vi "AH2700 Time Test.vi"() -> ()   [LabVIEW 2020]
uses:
  New NML Data Acq/Sub Controls/Instrument Properties.ctl
  New NML Data Acq/Sub Controls/Public.ctl
  New NML Data Acq/Sub Controls/Private.ctl
  New NML Data Acq/Sub Controls/Instrument Ref.ctl
  New NML Data Acq/Sub Controls/SystemCheckBox-resize.ctl
  New NML Data Acq/Sub Controls/Instrument Actions.ctl
  <vilib>/Analysis/NI_AALBase.lvlib
panel:
  out "Histogram Graph":T1(graph)
  out "Freq Index":i32
  out "Data":dbl[](array[numeric]) format="%_10f"
  out "Current Stats":dbl[](array[numeric]) format="%.3f"
  in  "Expected Value":dbl=100.0
  out "Count":i32
  out "Average":i32
  out "Current Frequency":dbl
  out "Array":dbl[][][](array[numeric])=[[[35.680109375, 0.6458252040579002, 35.498, 38.6, 64.0], [35.632625000000004, 0.528468752361218, 35.498, 38.549, 64.0], [35.539093750000006, 0.02657825746434977, 35.497, 35.656, 64.0], [36.008609375000006, 1.1004477100027956, 35.498, 38.6, 64.0], [36.059421875, 1.1460347899742611, 35.499, 38.599, 64.0], [36.01325000000001, 1.1049814334431005, 35.498, 38.601, 64.0], [36.20160937500001, 1.262523293730576, 35.498, 38.709, 64.0], [36.203921875, 1.2531691293737954, 35.498, 38.598, 64.0], [45.552343750000006, 1.1118567656231204, 45.047, 48.151, 64.0], [64.67654687500001, 1.1525081403794388, 64.1, 67.201, 64.0], [102.92346875000004, 1.2293001489265316, 102.249, 105.352, 64.0], [182.00240624999998, 0.9997699690786006, 181.55, 184.701, 64.0], [335.19457812499996, 1.4212888383624092, 334.149, 337.405, 64.0], [640.2555937499998, 1.285364116391284, 639.352, 642.698, 64.0], [1250.9235312499995, 1.329125825242058, 1249.751, 1253.499, 64.0], [2474.9906874999997, 1.2232058435579556, 2473.851, 2477.898, 64.0]], [[34.15467187499999, 1.2112240044837705, 33.349, 36.899, 64.0], [34.137171875, 1.2380397531208522, 33.349, 36.9, 64.0], [34.290296875, 1.3852482635744803, 33.347, 36.902, 64.0], [34.474890625, 1.2692667564221218, 33.347, 36.899, 64.0], [34.287546875000004, 1.3042409813567422, 33.348, 36.9, 64.0], [34.42039062500001, 1.3693168105043347, 33.347, 36.901, 64.0], [34.859515625, 1.4357561250245938, 33.348, 36.9, 64.0], [34.409515625000004, 1.38711379000378, 33.347, 36.9, 64.0], [43.403156249999995, 1.312365176370812, 42.399, 45.951, 64.0], [61.656375, 1.3327292738813536, 60.55, 64.15, 64.0], [98.21567187499998, 1.4193065046412856, 96.85, 100.601, 64.0], [173.53993749999998, 1.4269995258672636, 172.249, 175.851, 64.0], [318.38918749999993, 1.3004074193687212, 317.35, 321.052, 64.0], [609.0055312500001, 1.3376146023443207, 607.85, 611.599, 64.0], [1189.589046875, 1.035762834128312, 1188.749, 1192.4, 64.0], [2354.58440625, 1.292604946078635, 2353.049, 2357.304, 64.0]], [[34.75109375000001, 0.33744698437221915, 32.101, 34.921, 64.0], [34.712625, 0.47329498503274114, 32.1, 34.908, 64.0], [34.79143750000001, 0.02651676618460264, 34.748, 34.904, 64.0], [34.796265625, 0.021375139236528, 34.75, 34.911, 64.0], [34.795375, 0.028151799401171303, 34.748, 34.955, 64.0], [34.79615625000001, 0.022587550124680004, 34.749, 34.904, 64.0], [34.796921874999995, 0.025438568822364106, 34.749, 34.954, 64.0], [34.639984375000004, 0.6694339587657692, 32.051, 35.448, 64.0], [43.42746875, 0.6550800258577406, 40.899, 43.71, 64.0], [61.212609374999985, 0.029894851278045725, 61.148, 61.355, 64.0], [96.28523437499999, 0.6603404062549382, 93.749, 96.555, 64.0], [169.3985625, 0.6514420603065991, 166.899, 169.709, 64.0], [310.4539375, 0.07490520464253225, 310.3, 310.701, 64.0], [592.28128125, 0.06330286704557714, 592.101, 592.4, 64.0], [1155.7351875000002, 0.6178266535279325, 1153.301, 1156.301, 64.0], [2285.9500468749998, 0.3492272389641416, 2284.099, 2286.65, 64.0]], [[22.389156250000006, 0.026679888835112388, 22.347, 22.507, 64.0], [22.38890625000001, 0.0254238475414227, 22.347, 22.49, 64.0], [22.3896875, 0.029155780281267054, 22.347, 22.541, 64.0], [22.374859375000007, 0.08089830323480102, 21.95, 22.49, 64.0], [22.381375000000006, 0.06112061975086742, 21.949, 22.509, 64.0], [22.389921875000006, 0.025948853653916363, 22.348, 22.506, 64.0], [22.389156250000006, 0.026304818045007186, 22.347, 22.505, 64.0], [22.390671875, 0.025355913926177833, 22.348, 22.504, 64.0], [27.756406250000005, 0.025326263894564844, 27.7, 27.909, 64.0], [38.48835937500001, 0.026896844204750057, 38.448, 38.607, 64.0], [59.946937499999976, 0.07976928537281043, 59.499, 60.053, 64.0], [104.645328125, 0.06465538799225248, 104.201, 104.802, 64.0], [190.512546875, 0.03926625825945579, 190.448, 190.605, 64.0], [362.23907812500005, 0.0591844854958851, 362.102, 362.455, 64.0], [705.7094218749999, 0.0946466787563285, 705.449, 705.95, 64.0], [1394.2602031249999, 0.1881717536692792, 1393.899, 1394.75, 64.0]], [[20.119749999999996, 0.029883371178899207, 20.098, 20.262, 64.0], [20.118015624999998, 0.029038831247797867, 20.098, 20.254, 64.0], [20.119578125, 0.029699983799631628, 20.098, 20.255, 64.0], [20.121171874999998, 0.030004525948278734, 20.098, 20.256, 64.0], [20.12115625, 0.02950341317354455, 20.098, 20.254, 64.0], [20.118812499999994, 0.029183532538549214, 20.098, 20.253, 64.0], [20.121234374999997, 0.029925697502844035, 20.098, 20.26, 64.0], [20.11967187499999, 0.02985470353918612, 20.097, 20.26, 64.0], [25.024343749999996, 0.030163690329362818, 24.998, 25.156, 64.0], [34.832078125, 0.029021778733789375, 34.797, 34.954, 64.0], [54.45631249999998, 0.023024400445462147, 54.4, 54.553, 64.0], [95.23209375, 0.03525135086908385, 95.198, 95.404, 64.0], [173.71884375000002, 0.03747770501265849, 173.649, 173.807, 64.0], [330.65318749999994, 0.07354490583720144, 330.5, 330.803, 64.0], [644.43759375, 0.08689561677257476, 644.199, 644.658, 64.0], [1273.8344218750003, 0.2717127804676283, 1273.399, 1274.5, 64.0]], [[18.921562500000007, 0.02916775508173293, 18.888, 19.045, 64.0], [18.92150000000001, 0.028069641285644972, 18.898, 19.029, 64.0], [18.920703125000006, 0.027607613217003904, 18.898, 19.026, 64.0], [18.919921875000007, 0.027401949118196052, 18.898, 19.027, 64.0], [18.919734375000004, 0.030007534602771262, 18.898, 19.063, 64.0], [18.919671875, 0.029895083572811884, 18.898, 19.059, 64.0], [18.922000000000004, 0.030370202606324805, 18.898, 19.061, 64.0], [18.922859375000005, 0.030409306839524218, 18.898, 19.065, 64.0], [23.59, 0.027528916975450828, 23.548, 23.708, 64.0], [32.920515625, 0.03006289290407536, 32.898, 33.063, 64.0], [51.586828125, 0.027497506200057656, 51.548, 51.708, 64.0], [90.39075000000003, 0.036751849105840804, 90.348, 90.509, 64.0], [165.07832812500004, 0.041492035834583225, 164.998, 165.215, 64.0], [314.43070312500015, 0.05431614676689691, 314.348, 314.563, 64.0], [613.248578125, 0.12163043226746312, 613.048, 613.698, 64.0], [1212.055546875, 0.14712827031738435, 1211.749, 1212.35, 64.0]], [[17.816656249999998, 0.0295286886329374, 17.798, 17.965, 64.0], [17.817718749999997, 0.027549936623094604, 17.798, 17.934, 64.0], [17.817734374999993, 0.027530786338726063, 17.798, 17.935, 64.0], [17.81534375, 0.026946872333750548, 17.797, 17.935, 64.0], [17.815828124999996, 0.029024649998573397, 17.797, 17.962, 64.0], [17.815812499999996, 0.028893276528829944, 17.798, 17.962, 64.0], [17.81584375, 0.02919024557121701, 17.798, 17.963, 64.0], [17.818875, 0.02945402659297535, 17.798, 17.96, 64.0], [22.257953124999997, 0.023033743148101055, 22.201, 22.36, 64.0], [31.12675, 0.030695121374421677, 31.098, 31.263, 64.0], [48.867406249999995, 0.029459533046225145, 48.846, 49.013, 64.0], [85.71968749999999, 0.03148538335608076, 85.649, 85.863, 64.0], [156.70874999999998, 0.040979669756274886, 156.648, 156.859, 64.0], [298.70846875, 0.06911273715103122, 298.552, 298.989, 64.0], [582.6431093749999, 0.09314029649592803, 582.451, 582.851, 64.0], [1151.900953125, 0.16111480966951955, 1151.549, 1152.201, 64.0]], [[12.034593749999997, 0.028898683855349418, 11.998, 12.164, 64.0], [12.032890624999997, 0.028826859822433472, 11.998, 12.154, 64.0], [12.033609374999997, 0.02827170731533241, 11.998, 12.15, 64.0], [12.032124999999999, 0.029193117257978757, 11.998, 12.158, 64.0], [12.033828124999998, 0.02916812496354362, 11.999, 12.164, 64.0], [12.032171875, 0.029296814219513724, 11.998, 12.157, 64.0], [12.033703124999997, 0.028648210940290315, 11.999, 12.158, 64.0], [12.034593749999997, 0.0289760266262926, 11.998, 12.165, 64.0], [18.054062499999993, 0.019095312314308017, 17.999, 18.157, 64.0], [23.690781250000008, 0.028795650437643813, 23.648, 23.81, 64.0], [37.69114062499999, 0.02669157597772372, 37.649, 37.785, 64.0], [61.56656250000001, 0.030213460156082395, 61.502, 61.709, 64.0], [103.91493750000002, 0.036512609259276095, 103.848, 104.008, 64.0], [194.06262499999997, 0.048098279017490406, 193.949, 194.158, 64.0], [377.20871875, 0.21695939703160655, 375.698, 377.5, 64.0], [736.31140625, 0.1294840455637457, 736.051, 736.651, 64.0]], [[10.913875, 0.026392940374033676, 10.897, 11.04, 64.0], [10.91528125, 0.026391117282687622, 10.898, 11.027, 64.0], [10.913687500000002, 0.025685444584278988, 10.898, 11.026, 64.0], [10.912625000000002, 0.024161822174530907, 10.897, 11.009, 64.0], [10.913406249999996, 0.027790439574537692, 10.897, 11.059, 64.0], [10.915812499999996, 0.02584991787159579, 10.898, 11.011, 64.0], [10.914171874999997, 0.02808747938167244, 10.898, 11.059, 64.0], [10.912640625, 0.027903670571256627, 10.897, 11.06, 64.0], [16.703343750000002, 0.02255308992309843, 16.65, 16.813, 64.0], [21.878234374999998, 0.029866232026758453, 21.848, 22.007, 64.0], [32.232125, 0.030629117798964347, 32.198, 32.358, 64.0], [56.71710937499999, 0.028554663360004038, 56.697, 56.848, 64.0], [95.565765625, 0.034891551798460964, 95.498, 95.661, 64.0], [180.93056249999998, 0.05610106384980118, 180.799, 181.056, 64.0], [343.9290156249999, 0.1001364929099364, 343.65, 344.148, 64.0], [676.3548124999999, 0.11533950919330764, 676.149, 676.75, 64.0]], [[9.85490625, 0.01860339510744764, 9.847, 9.965, 64.0], [9.859046875000002, 0.023257993804144908, 9.847, 9.98, 64.0], [9.856703125000001, 0.021655073592615207, 9.847, 9.982, 64.0], [9.857218749999998, 0.0211183127858414, 9.847, 9.967, 64.0], [9.856406249999997, 0.020395859173581478, 9.847, 9.965, 64.0], [9.855687499999998, 0.019493486905785416, 9.847, 9.967, 64.0], [9.857203125000003, 0.020914170549220915, 9.848, 9.964, 64.0], [9.855625000000002, 0.018946457557238776, 9.847, 9.961, 64.0], [15.229812500000003, 0.029802458085475266, 15.196, 15.36, 64.0], [20.366484375000002, 0.02894164472871517, 20.348, 20.509, 64.0], [30.6329375, 0.029038493882846485, 30.598, 30.758, 64.0], [52.392328124999985, 0.02657248528471503, 52.348, 52.511, 64.0], [93.45318749999998, 0.03566060251073456, 93.398, 93.557, 64.0], [176.92834374999998, 0.05984244359612746, 176.799, 177.053, 64.0], [339.8040468749999, 0.07102725380957979, 339.649, 339.999, 64.0], [669.5345156249999, 0.09183629192149022, 669.3, 669.75, 64.0]], [[5.317374999999999, 0.055725090527389165, 5.05, 5.513, 64.0], [5.275406249999999, 0.12404335119703305, 4.997, 5.426, 64.0], [5.28784375, 0.10080772500475807, 5.047, 5.403, 64.0], [5.2751875, 0.11921847025857052, 5.0, 5.511, 64.0], [5.31890625, 0.07831230087447293, 5.0, 5.411, 64.0], [5.2947187499999995, 0.11687144867705292, 5.0, 5.51, 64.0], [5.31578125, 0.0728051255717879, 5.049, 5.409, 64.0], [5.320437499999998, 0.08153251858799403, 5.0, 5.46, 64.0], [6.464281250000001, 0.1146490114799658, 6.199, 6.712, 64.0], [8.822718749999998, 0.10587420939154965, 8.548, 8.952, 64.0], [13.504781250000002, 0.11398878652034582, 13.247, 13.658, 64.0], [23.254796874999993, 0.0951271796467217, 22.948, 23.548, 64.0], [42.04464062500001, 0.08548598087749393, 41.749, 42.258, 64.0], [79.58610937499998, 0.09248854363846871, 79.299, 79.759, 64.0], [154.7024375, 0.08006284733763569, 154.401, 154.857, 64.0], [305.17040625, 0.17328916275569853, 304.699, 305.602, 64.0]], [[4.787750000000002, 0.02803399297111919, 4.748, 4.917, 64.0], [4.787218749999998, 0.02942705199113371, 4.747, 4.933, 64.0], [4.787218749999999, 0.029322762570431666, 4.748, 4.932, 64.0], [4.786890625, 0.02771688911945777, 4.747, 4.909, 64.0], [4.786796874999998, 0.027499021447236194, 4.748, 4.907, 64.0], [4.786015625, 0.027576440478140854, 4.748, 4.905, 64.0], [4.786875, 0.02786048006058671, 4.747, 4.91, 64.0], [4.787609375000001, 0.027541378501482184, 4.747, 4.908, 64.0], [5.949343750000001, 0.01979756177868758, 5.898, 6.06, 64.0], [8.275203125, 0.030368205850647603, 8.248, 8.412, 64.0], [13.60240625, 0.024902169695742517, 13.547, 13.755, 64.0], [23.221921875000003, 0.029635513170400803, 23.198, 23.352, 64.0], [41.12589062500001, 0.03024404293305624, 41.097, 41.26, 64.0], [78.29778125000001, 0.04687858980963104, 78.248, 78.5, 64.0], [152.65714062499998, 0.04361951914449336, 152.547, 152.751, 64.0], [301.6712031250001, 0.06336845634794074, 301.549, 301.807, 64.0]], [[4.4963750000000005, 0.022037125961316323, 4.449, 4.619, 64.0], [4.495921875000001, 0.024482131279447983, 4.449, 4.637, 64.0], [4.4959218750000005, 0.02442241014035045, 4.449, 4.638, 64.0], [4.496265625, 0.021251511384160676, 4.45, 4.612, 64.0], [4.497, 0.020346209818250017, 4.449, 4.608, 64.0], [4.496249999999999, 0.021433544396502066, 4.448, 4.611, 64.0], [4.495453125, 0.022207484572363132, 4.448, 4.61, 64.0], [4.495515625000001, 0.022266775154782766, 4.448, 4.612, 64.0], [5.552468750000001, 0.019504959686729734, 5.499, 5.659, 64.0], [7.662671874999999, 0.027638858478885763, 7.646, 7.813, 64.0], [11.886078125000001, 0.028300151262986812, 11.847, 12.012, 64.0], [21.574796875, 0.02887695829269627, 21.547, 21.687, 64.0], [37.556453125, 0.029368987902153112, 37.501, 37.664, 64.0], [71.3338125, 0.03879775603067485, 71.251, 71.514, 64.0], [138.95717187499997, 0.04298192853462396, 138.852, 139.108, 64.0], [274.45556250000004, 0.06730453768989665, 274.298, 274.65, 64.0]], [[0.045796874999999994, 0.0009788183270966677, 0.044, 0.048, 64.0], [0.07882812500000003, 0.0023132104228360787, 0.074, 0.082, 64.0], [1.2261875, 0.04771837854321593, 1.149, 1.396, 64.0], [1.4296875, 0.0582051312307369, 1.349, 1.601, 64.0], [2.028171875, 0.07354915313303954, 1.848, 2.202, 64.0], [2.202765625, 0.0065725310712494815, 2.199, 2.253, 64.0], [3.0022968750000003, 0.018688490378279552, 2.997, 3.149, 64.0], [4.52203125, 0.026889526343617985, 4.498, 4.611, 64.0], [7.319671875000001, 0.024660266021235323, 7.298, 7.36, 64.0], [9.907234374999998, 0.017866117784301652, 9.897, 9.963, 64.0], [16.533578125, 0.025463203882939062, 16.497, 16.598, 64.0], [27.401546874999994, 0.017758458469760943, 27.347, 27.451, 64.0], [46.658656249999986, 0.024822684677591956, 46.599, 46.754, 64.0], [88.09312499999999, 0.041037922841086975, 88.048, 88.211, 64.0], [170.98215625, 0.04138177604802538, 170.9, 171.1, 64.0], [337.23678125000004, 0.06379791227862742, 337.099, 337.35, 64.0]], [[0.04460937499999999, 0.0022226624068002712, 0.039, 0.05, 64.0], [0.075875, 0.002200288581361511, 0.073, 0.082, 64.0], [1.2364375, 0.05530058554757592, 1.14, 1.357, 64.0], [1.445046875, 0.054552269877701, 1.348, 1.585, 64.0], [1.95403125, 0.07693967307995785, 1.798, 2.052, 64.0], [2.7555781250000004, 0.022627981475043704, 2.747, 2.906, 64.0], [2.9597812500000003, 0.023547634094077705, 2.948, 3.076, 64.0], [4.47128125, 0.027028772881728565, 4.448, 4.564, 64.0], [7.263437499999999, 0.02258730855893437, 7.248, 7.311, 64.0], [9.843906250000002, 0.01943382646601315, 9.798, 9.908, 64.0], [15.005609374999999, 0.016058046677452375, 14.998, 15.058, 64.0], [27.232859374999997, 0.02563533473361988, 27.198, 27.302, 64.0], [46.445546875000005, 0.02648505399876413, 46.398, 46.549, 64.0], [87.699328125, 0.04146295140587197, 87.648, 87.899, 64.0], [170.24621875000003, 0.06976092251055598, 170.1, 170.5, 64.0], [335.7454218750001, 0.07148311037891743, 335.551, 335.902, 64.0]], [[0.04279687499999999, 0.0009116475143805235, 0.041, 0.045, 64.0], [0.07453125000000001, 0.0017903511227848965, 0.07, 0.08, 64.0], [1.13803125, 0.04628310698368781, 1.08, 1.238, 64.0], [1.4262656249999996, 0.06696273357989548, 1.299, 1.551, 64.0], [1.9219843749999999, 0.08635410527598483, 1.749, 2.057, 64.0], [2.7156562500000003, 0.028373483457130606, 2.698, 2.853, 64.0], [3.5164687499999996, 0.02844765103143578, 3.497, 3.655, 64.0], [4.685671875, 0.026589205762775917, 4.647, 4.784, 64.0], [7.624375, 0.025285355570946782, 7.598, 7.661, 64.0], [10.194671875, 0.018587463506438362, 10.149, 10.259, 64.0], [15.3345625, 0.02561179973594774, 15.297, 15.412, 64.0], [26.105640625, 0.022871183218745043, 26.048, 26.16, 64.0], [46.674343750000006, 0.02669356901922447, 46.647, 46.748, 64.0], [87.78531250000002, 0.029304030277015447, 87.702, 87.853, 64.0], [169.98764062499998, 0.0643093632096331, 169.851, 170.201, 64.0], [334.9305625, 0.09108288132157924, 334.75, 335.2, 64.0]], [[0.04143749999999999, 0.000833333333333333, 0.04, 0.043, 64.0], [0.07156250000000004, 0.0022947490093413263, 0.068, 0.076, 64.0], [1.076640625, 0.019271961035215307, 1.064, 1.167, 64.0], [1.3071718749999999, 0.0381856595236218, 1.199, 1.407, 64.0], [1.8758750000000002, 0.061556142911643935, 1.702, 2.001, 64.0], [2.6616875000000007, 0.02638053334719638, 2.648, 2.8, 64.0], [3.46184375, 0.02707732534093881, 3.447, 3.609, 64.0], [4.631421874999999, 0.02970425905408825, 4.597, 4.763, 64.0], [7.5618437499999995, 0.021589399772566187, 7.548, 7.611, 64.0], [10.122812500000002, 0.02548630195421793, 10.098, 10.162, 64.0], [15.240015624999998, 0.022710386538895278, 15.198, 15.31, 64.0], [25.960218750000006, 0.020404223613502987, 25.948, 26.006, 64.0], [46.438406249999986, 0.026144724649231493, 46.398, 46.5, 64.0], [87.3485625, 0.031112634599886134, 87.297, 87.408, 64.0], [169.20246875000004, 0.06788271134832582, 169.098, 169.359, 64.0], [333.4696406250001, 0.11147330340054809, 333.249, 333.751, 64.0]], [[0.0394375, 0.0008886408384057875, 0.037, 0.041, 64.0], [0.060484375, 0.002960009585462816, 0.059, 0.083, 64.0], [0.41979687499999996, 0.4181574921534321, 0.067, 1.028, 64.0], [1.0312500000000002, 0.1205415030943864, 0.338, 1.25, 64.0], [1.1069843750000001, 0.07690305011547652, 0.996, 1.303, 64.0], [1.36771875, 0.010803392691686875, 1.351, 1.446, 64.0], [1.768046875, 0.029313537523520714, 1.748, 1.907, 64.0], [2.810296875, 0.026678378194621214, 2.798, 2.962, 64.0], [3.3626875, 0.028145807999354094, 3.347, 3.514, 64.0], [4.461093750000001, 0.026948344914869877, 4.447, 4.61, 64.0], [6.933703125000001, 0.056644723955405846, 6.75, 7.107, 64.0], [11.458687500000002, 0.0638805619142176, 11.299, 11.609, 64.0], [20.294687500000002, 0.06133537134295151, 20.048, 20.459, 64.0], [37.856359375, 0.07883282838608044, 37.649, 38.059, 64.0], [73.3368125, 0.2120888459382737, 72.849, 73.699, 64.0], [144.37354687500002, 0.11099376926420693, 144.198, 144.65, 64.0]], [[0.03875, 0.0009258200997725524, 0.037, 0.041, 64.0], [0.05954687499999999, 0.0012463239597706572, 0.057, 0.062, 64.0], [0.28712500000000013, 0.36703010126976676, 0.067, 1.095, 64.0], [1.00884375, 0.2712667648977575, 0.124, 1.267, 64.0], [1.1458593749999997, 0.16141456703283263, 0.193, 1.39, 64.0], [1.4290156250000001, 0.06595609222195076, 1.348, 1.599, 64.0], [1.8261250000000002, 0.035505197473314355, 1.75, 1.97, 64.0], [2.9649531250000005, 0.10342107330122702, 2.849, 3.153, 64.0], [3.586109375, 0.07221267469706937, 3.351, 3.758, 64.0], [4.6891875, 0.067257589410663, 4.498, 4.859, 64.0], [6.893109375, 0.06736729864398082, 6.7, 7.058, 64.0], [11.409546875, 0.0711457100152315, 11.199, 11.561, 64.0], [20.20009375, 0.05858346880699643, 20.049, 20.354, 64.0], [37.74307812500002, 0.0814311092005688, 37.548, 37.905, 64.0], [72.81415625000001, 0.08406143232637607, 72.599, 73.0, 64.0], [143.122, 0.09146080780902453, 142.949, 143.349, 64.0]], [[0.039203125000000005, 0.0035642835273715346, 0.036, 0.058, 64.0], [0.05773437499999999, 0.0028241711103113892, 0.056, 0.079, 64.0], [0.21651562500000004, 0.3235569669518727, 0.066, 1.019, 64.0], [0.8624843750000002, 0.3220957657152088, 0.121, 1.176, 64.0], [1.0681875, 0.13232798058024028, 0.17, 1.224, 64.0], [1.4196093750000003, 0.06044901227743477, 1.348, 1.655, 64.0], [1.7612968750000002, 0.041348568500777526, 1.698, 1.881, 64.0], [2.8438593749999996, 0.10782037784652888, 2.598, 3.058, 64.0], [3.3517656250000005, 0.09153709321648688, 3.147, 3.563, 64.0], [4.370421875000002, 0.08218558261690044, 4.101, 4.61, 64.0], [6.350249999999999, 0.08515066013035323, 6.099, 6.517, 64.0], [10.428984374999999, 0.10589564977312817, 10.199, 10.557, 64.0], [18.411140625000005, 0.08429876332435662, 18.198, 18.563, 64.0], [34.31735937500001, 0.09803099075705364, 34.098, 34.511, 64.0], [66.18135937500001, 0.09176909726210403, 65.95, 66.307, 64.0], [129.93446875, 0.13216199400254997, 129.598, 130.202, 64.0]], [[0.037718749999999995, 0.0025289984842489202, 0.035, 0.056, 64.0], [0.05610937500000001, 0.0008929563436954983, 0.054, 0.059, 64.0], [0.375171875, 0.3829513025814242, 0.063, 0.98, 64.0], [0.7453281250000001, 0.330907269161211, 0.12, 1.116, 64.0], [1.0157812499999999, 0.04729222519074423, 0.949, 1.158, 64.0], [1.3915156250000007, 0.035751342382389716, 1.348, 1.557, 64.0], [1.7426562500000007, 0.019440767792989855, 1.732, 1.837, 64.0], [2.8056562499999997, 0.08329641444101997, 2.648, 3.012, 64.0], [3.318906249999999, 0.07777577024053142, 3.15, 3.509, 64.0], [4.331390625, 0.0584673609090291, 4.149, 4.46, 64.0], [6.317328125000001, 0.06414345398005986, 6.148, 6.511, 64.0], [10.397765625000002, 0.07064009882147612, 10.248, 10.559, 64.0], [18.328218749999998, 0.06959211521429691, 18.151, 18.51, 64.0], [34.24776562500001, 0.07327048003150806, 34.099, 34.408, 64.0], [66.00728125, 0.07893567176997879, 65.749, 66.265, 64.0], [129.650125, 0.11174624030463993, 129.451, 129.9, 64.0]], [[0.037265625000000004, 0.0033582033532686436, 0.034, 0.056, 64.0], [0.055125, 0.0013153549825650611, 0.053, 0.059, 64.0], [0.3305624999999999, 0.36865770569493594, 0.062, 0.934, 64.0], [0.6878281249999999, 0.3780662810238732, 0.11, 1.072, 64.0], [0.97025, 0.07404245886169444, 0.797, 1.104, 64.0], [1.1524375000000002, 0.06645439419584312, 1.012, 1.254, 64.0], [1.6931406249999998, 0.04386590938248495, 1.648, 1.861, 64.0], [2.5013906250000004, 0.05567639412798958, 2.447, 2.65, 64.0], [3.3001250000000013, 0.07594954465520734, 3.149, 3.46, 64.0], [4.307953125, 0.07052151077609481, 4.147, 4.497, 64.0], [6.278281250000001, 0.07787178488356604, 6.099, 6.46, 64.0], [10.364234375, 0.072844854093183, 10.198, 10.562, 64.0], [18.28145312499999, 0.07622521552703451, 18.1, 18.414, 64.0], [34.121281249999996, 0.07735538863449484, 33.948, 34.363, 64.0], [65.7501875, 0.0868470421497402, 65.552, 65.951, 64.0], [129.661734375, 0.30290221808404993, 129.049, 130.15, 64.0]], [[0.0360625, 0.0009236745114890851, 0.034, 0.038, 64.0], [0.0545, 0.0008164965809277267, 0.052, 0.058, 64.0], [0.3715625, 0.3776916469273978, 0.061, 0.924, 64.0], [0.6041562500000001, 0.3981545212822031, 0.108, 1.107, 64.0], [0.9742499999999998, 0.05337676802766691, 0.821, 1.104, 64.0], [1.123375, 0.05925181666225751, 0.993, 1.259, 64.0], [1.6516562499999998, 0.04798121945756401, 1.598, 1.91, 64.0], [2.490578125, 0.06359764513148145, 2.398, 2.697, 64.0], [3.276671875, 0.05685376805859325, 3.198, 3.407, 64.0], [4.23925, 0.03799122705748434, 4.15, 4.412, 64.0], [6.217249999999997, 0.046761807778000486, 6.1, 6.407, 64.0], [10.30246875, 0.05330653158407341, 10.199, 10.461, 64.0], [18.257187499999997, 0.0633012136597211, 18.099, 18.409, 64.0], [34.168875, 0.07139283232885828, 34.048, 34.361, 64.0], [65.95253125, 0.0806457998886651, 65.8, 66.262, 64.0], [129.76103125, 0.127245665251894, 129.447, 130.099, 64.0]], [[0.035859375000000006, 0.0010520907001156494, 0.034, 0.038, 64.0], [0.052765625, 0.0009384585047189705, 0.05, 0.055, 64.0], [0.4195781249999999, 0.36543363259468775, 0.061, 0.919, 64.0], [0.1475, 0.1706273206133254, 0.106, 0.968, 64.0], [0.973921875, 0.09009594615679935, 0.81, 1.238, 64.0], [1.16875, 0.11702774057244744, 0.939, 1.539, 64.0], [1.595375, 0.03213142653895982, 1.548, 1.754, 64.0], [2.422062500000001, 0.04284222624008175, 2.348, 2.663, 64.0], [3.268859375, 0.06570759352785811, 3.099, 3.462, 64.0], [4.214921875, 0.07571150437576366, 4.05, 4.362, 64.0], [6.224984375, 0.10113380923821544, 5.999, 6.4, 64.0], [10.257890625000002, 0.08681601000537849, 10.198, 10.557, 64.0], [18.185140625000003, 0.0801658731150706, 18.099, 18.451, 64.0], [34.15160937500001, 0.46394538598907914, 33.949, 37.75, 64.0], [65.817296875, 0.05896183314532537, 65.748, 66.009, 64.0], [129.46579687500002, 0.07363534772460643, 129.3, 129.75, 64.0]], [[0.03492187500000001, 0.0008223984956906737, 0.033, 0.037, 64.0], [0.048859375000000003, 0.000906190132122148, 0.047, 0.051, 64.0], [0.4915312499999999, 0.4735709989763188, 0.053, 1.128, 64.0], [0.4984687499999999, 0.40133230377774914, 0.094, 0.979, 64.0], [0.8445937500000001, 0.30391141768875235, 0.125, 1.276, 64.0], [0.983515625, 0.08167220431905418, 0.826, 1.376, 64.0], [1.1046562500000001, 0.052486799171806875, 0.999, 1.25, 64.0], [1.7495312500000002, 0.030927959688220475, 1.65, 1.924, 64.0], [2.4446875, 0.032039596038116874, 2.35, 2.614, 64.0], [2.9298125, 0.04775861095797196, 2.798, 3.11, 64.0], [3.8899218750000006, 0.05683484977379214, 3.798, 4.061, 64.0], [5.964937499999998, 0.041770679699278106, 5.849, 6.106, 64.0], [9.878250000000001, 0.04334688432808478, 9.798, 10.061, 64.0], [17.732796875000002, 0.03278606928690462, 17.649, 17.859, 64.0], [33.396890625000005, 0.04579287987473907, 33.299, 33.557, 64.0], [64.81414062500001, 0.052618684347485116, 64.65, 64.961, 64.0]], [[0.034562499999999996, 0.0008886408384057861, 0.033, 0.038, 64.0], [0.32259375, 0.4921232172055068, 0.036, 1.306, 58.0], [0.482453125, 0.4753202739703223, 0.051, 1.306, 61.0], [0.491140625, 0.4012747096555264, 0.09, 1.12, 64.0], [0.5685781249999999, 0.38575338798160375, 0.125, 1.038, 64.0], [0.9647968750000001, 0.07795627176526392, 0.777, 1.113, 64.0], [1.12715625, 0.11359063491886046, 0.908, 1.519, 64.0], [1.7391874999999999, 0.031040615993724114, 1.696, 1.909, 64.0], [2.4188437500000006, 0.05083250389643374, 2.347, 2.549, 64.0], [2.926640625, 0.05148997966548813, 2.848, 3.158, 64.0], [3.88290625, 0.05199472462557032, 3.799, 4.063, 64.0], [5.942312500000002, 0.05193123505755636, 5.848, 6.111, 64.0], [9.868812499999999, 0.047211740199852865, 9.751, 10.009, 64.0], [17.697687500000004, 0.03771441347982217, 17.599, 17.858, 64.0], [33.336828125, 0.03784452516966645, 33.248, 33.511, 64.0], [64.647703125, 0.07144310194466734, 64.498, 64.86, 64.0]], [[0.034296875, 0.0008485222916135317, 0.032, 0.036, 64.0], [0.29162499999999997, 0.4902076819354949, 0.019, 1.307, 50.0], [0.4726249999999999, 0.4397943061773672, 0.051, 1.306, 63.0], [0.6356562499999998, 0.36883218616007346, 0.091, 1.132, 64.0], [0.41043750000000007, 0.372063993258371, 0.124, 0.987, 64.0], [0.9902343750000001, 0.14060410955942934, 0.818, 1.54, 64.0], [1.1521406250000001, 0.20133647641724317, 0.94, 1.931, 64.0], [1.7434375000000002, 0.03018928381301645, 1.697, 1.881, 64.0], [2.4345625, 0.03728435349946436, 2.352, 2.612, 64.0], [2.9250624999999997, 0.03710383328504545, 2.848, 3.061, 64.0], [3.901640625, 0.038244562716560807, 3.8, 4.058, 64.0], [5.93765625, 0.04446193976089653, 5.849, 6.113, 64.0], [9.798625, 0.044017492915200115, 9.748, 9.914, 64.0], [17.644671875, 0.04819637564174316, 17.548, 17.748, 64.0], [33.314937500000006, 0.03791128951929587, 33.25, 33.46, 64.0], [64.61264062500001, 0.05483781778955678, 64.4, 64.813, 64.0]], [[0.034156249999999985, 0.0009295629626804749, 0.032, 0.037, 64.0], [0.37470312499999997, 0.536750826872963, 0.025, 1.306, 52.0], [0.36146875, 0.4369580259799034, 0.05, 1.305, 63.0], [0.41892187499999994, 0.3951386457373649, 0.089, 1.25, 64.0], [0.5661875000000001, 0.42557840659357965, 0.027, 1.316, 63.0], [1.0445625, 0.16097164050732368, 0.77, 1.588, 64.0], [1.165859375, 0.21122611574851805, 0.963, 2.11, 64.0], [1.7286249999999999, 0.03152147164399489, 1.698, 1.882, 64.0], [2.4290468750000005, 0.039535569553512645, 2.349, 2.612, 64.0], [2.9220468749999995, 0.034130203394210246, 2.85, 3.063, 64.0], [3.8923125, 0.0427383605244452, 3.797, 4.06, 64.0], [5.923625000000001, 0.051874543409732875, 5.8, 6.113, 64.0], [9.847796875000002, 0.028209071876102297, 9.749, 9.962, 64.0], [17.668843750000008, 0.0502600282183362, 17.549, 17.807, 64.0], [33.28292187500001, 0.05041016044205417, 33.147, 33.457, 64.0], [64.524328125, 0.1156377835061112, 64.349, 64.756, 64.0]], [[0.03425000000000001, 0.0009594972228385659, 0.032, 0.037, 64.0], [0.34709375, 0.5246204287349395, 0.018, 1.306, 53.0], [0.5341250000000001, 0.4468221655413344, 0.052, 1.305, 63.0], [0.40681249999999997, 0.38798133955290925, 0.09, 0.986, 64.0], [0.526734375, 0.3948829138175011, 0.123, 1.257, 64.0], [1.0065625, 0.12163683587330706, 0.85, 1.319, 64.0], [1.121359375, 0.09203404601015865, 0.918, 1.47, 64.0], [1.6511093749999999, 0.03285374863852182, 1.596, 1.772, 64.0], [2.3540312500000002, 0.03785434438593392, 2.298, 2.561, 64.0], [2.8376562499999993, 0.036328841465455855, 2.798, 3.011, 64.0], [3.811, 0.030756080828618436, 3.798, 3.958, 64.0], [5.875125000000001, 0.04570627409955327, 5.799, 6.007, 64.0], [9.797015625, 0.046804046829341375, 9.699, 9.913, 64.0], [17.648531250000005, 0.03464054361445198, 17.552, 17.749, 64.0], [33.214968750000004, 0.07158898752546078, 33.099, 33.409, 64.0], [64.52198437499999, 0.05583066580337122, 64.4, 64.7, 64.0]], [[0.03434374999999999, 0.0010113443826498764, 0.031, 0.037, 64.0], [0.047359375, 0.0008612871043911417, 0.046, 0.05, 64.0], [0.6163437500000001, 0.449449017846137, 0.05, 1.305, 63.0], [0.20310937499999998, 0.2660311544703167, 0.088, 0.926, 64.0], [0.587796875, 0.3999974674398993, 0.121, 1.284, 64.0], [0.971921875, 0.11584873891216808, 0.725, 1.25, 64.0], [1.1726249999999996, 0.19083779366798262, 0.932, 2.172, 64.0], [1.695453125, 0.04207058682492619, 1.597, 1.81, 64.0], [2.3853281250000005, 0.045926115504334356, 2.296, 2.511, 64.0], [2.8728593750000004, 0.04918215807199852, 2.798, 3.012, 64.0], [3.845359375, 0.046197425609404985, 3.798, 4.005, 64.0], [5.896999999999999, 0.04625979089844934, 5.8, 6.011, 64.0], [9.801703125, 0.045940154199318343, 9.699, 9.957, 64.0], [17.573562499999998, 0.04523444220839678, 17.499, 17.754, 64.0], [33.149328125000004, 0.06713787157486586, 33.049, 33.352, 64.0], [64.41103125, 0.07505151008918137, 64.249, 64.658, 64.0]], [[0.034249999999999996, 0.0018430478552727263, 0.032, 0.047, 64.0], [0.32334375000000004, 0.5052640114139921, 0.046, 1.306, 57.0], [0.4938593749999999, 0.4588160009937068, 0.05, 1.125, 64.0], [0.246859375, 0.2997355377814366, 0.089, 0.978, 64.0], [0.655328125, 0.39092422253917336, 0.123, 1.259, 64.0], [0.9609531250000001, 0.10345790182676637, 0.762, 1.235, 64.0], [1.1225781250000002, 0.17450836198525782, 0.893, 1.81, 64.0], [1.6698281249999998, 0.048324155019341355, 1.6, 1.802, 64.0], [2.38684375, 0.048502076129676004, 2.297, 2.558, 64.0], [2.8588281249999996, 0.04393449477744343, 2.798, 3.001, 64.0], [3.823562500000001, 0.06400468112840814, 3.747, 4.161, 64.0], [5.859453125, 0.051471036604356264, 5.797, 6.05, 64.0], [9.766531250000003, 0.050006973720021476, 9.698, 9.907, 64.0], [17.554078125, 0.04870100050714412, 17.498, 17.701, 64.0], [33.148546875, 0.0650579545512835, 33.048, 33.301, 64.0], [64.35553125, 0.07546637404242508, 64.198, 64.607, 64.0]], [[0.034515625, 0.0008907315969346642, 0.033, 0.037, 64.0], [0.3649374999999999, 0.5362591139566648, 0.038, 1.306, 53.0], [0.6037968750000001, 0.4594191702120552, 0.05, 1.093, 64.0], [0.4445781250000001, 0.3924431332654736, 0.089, 1.25, 64.0], [0.665234375, 0.4321997900070555, 0.049, 1.306, 60.0], [0.9970937499999999, 0.15715786409222973, 0.741, 1.337, 64.0], [1.2488281249999997, 0.2925134404556861, 0.89, 2.037, 64.0], [1.7253124999999998, 0.04695383582214233, 1.697, 1.922, 64.0], [2.418109375, 0.035445069143497265, 2.397, 2.561, 64.0], [2.9307343749999997, 0.05072216327427515, 2.849, 3.116, 64.0], [3.9001406249999997, 0.049276952076527464, 3.799, 4.009, 64.0], [5.9368125, 0.04772103958473263, 5.849, 6.099, 64.0], [9.82353125, 0.050169227509389444, 9.749, 9.96, 64.0], [17.583671875, 0.039226673257380315, 17.499, 17.706, 64.0], [33.10329687500001, 0.05189203678930808, 33.049, 33.362, 64.0], [64.258703125, 0.07296719847692917, 64.148, 64.45, 64.0]], [[0.034140624999999994, 0.0008885012795767511, 0.032, 0.037, 64.0], [0.047468750000000004, 0.0010685808717009124, 0.045, 0.05, 64.0], [0.5396093749999998, 0.5011319129694581, 0.05, 1.306, 56.0], [0.5432187500000001, 0.43437839070276485, 0.089, 1.26, 64.0], [0.7524687500000001, 0.31857111382467196, 0.122, 1.17, 64.0], [1.035640625, 0.14474754894846165, 0.802, 1.346, 64.0], [1.25265625, 0.21314941616413383, 0.866, 1.855, 64.0], [1.7620156250000003, 0.038871171913802384, 1.699, 1.923, 64.0], [2.4587343749999997, 0.03657574970208873, 2.399, 2.609, 64.0], [2.9595624999999997, 0.034324259087484474, 2.899, 3.114, 64.0], [3.929046875, 0.029809676540952155, 3.897, 4.059, 64.0], [5.93915625, 0.03864622561089572, 5.853, 6.057, 64.0], [9.826687499999998, 0.0301387663665127, 9.796, 9.959, 64.0], [17.576703124999998, 0.035961036978312926, 17.5, 17.71, 64.0], [33.071234374999996, 0.03920185539320605, 32.998, 33.208, 64.0], [64.17823437499999, 0.04647810277645133, 64.051, 64.356, 64.0]]] format="%.3g"
  in  "# Calls":i32=64
  out "Data":dbl[](array[numeric]) format="%_10f"
  # "Average"
  # "Std Dev"
  # "Min"
  # "Max"
  # "# Valid"
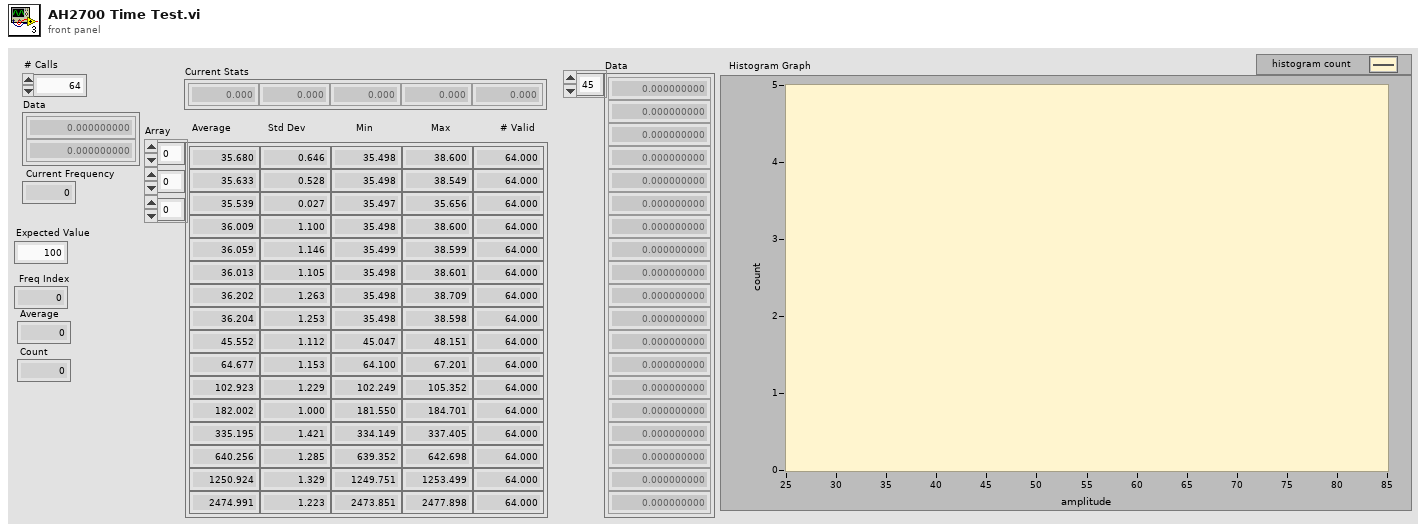
[diagram p1: front panel]
types:
  T1 = cluster{"X Values":dbl[], "Histogram: h(x)":i32[]}
  T2 = typedef "Instrument Properties.ctl" = cluster{"Public":T3, "Private":T4}
  T3 = typedef "Public.ctl" = cluster{"Column Name":string[], "Trace Color":u32[]}
  T4 = typedef "Private.ctl" = cluster{"Path":path, "VI Refnum":T5, "Name":string, "# of Values":i32, "Scale Factors":dbl[], "Display":T6[], "Offset":dbl[]}
  T5 = typedef "Instrument Ref.ctl" = refnum<vi>
  T6 = typedef "SystemCheckBox-resize.ctl" = bool
  T7 = typedef "Instrument Actions.ctl" = enum16{"Scan", "Identify", "New", "Configure", "Initialize", "Test", "Read", "Close"}
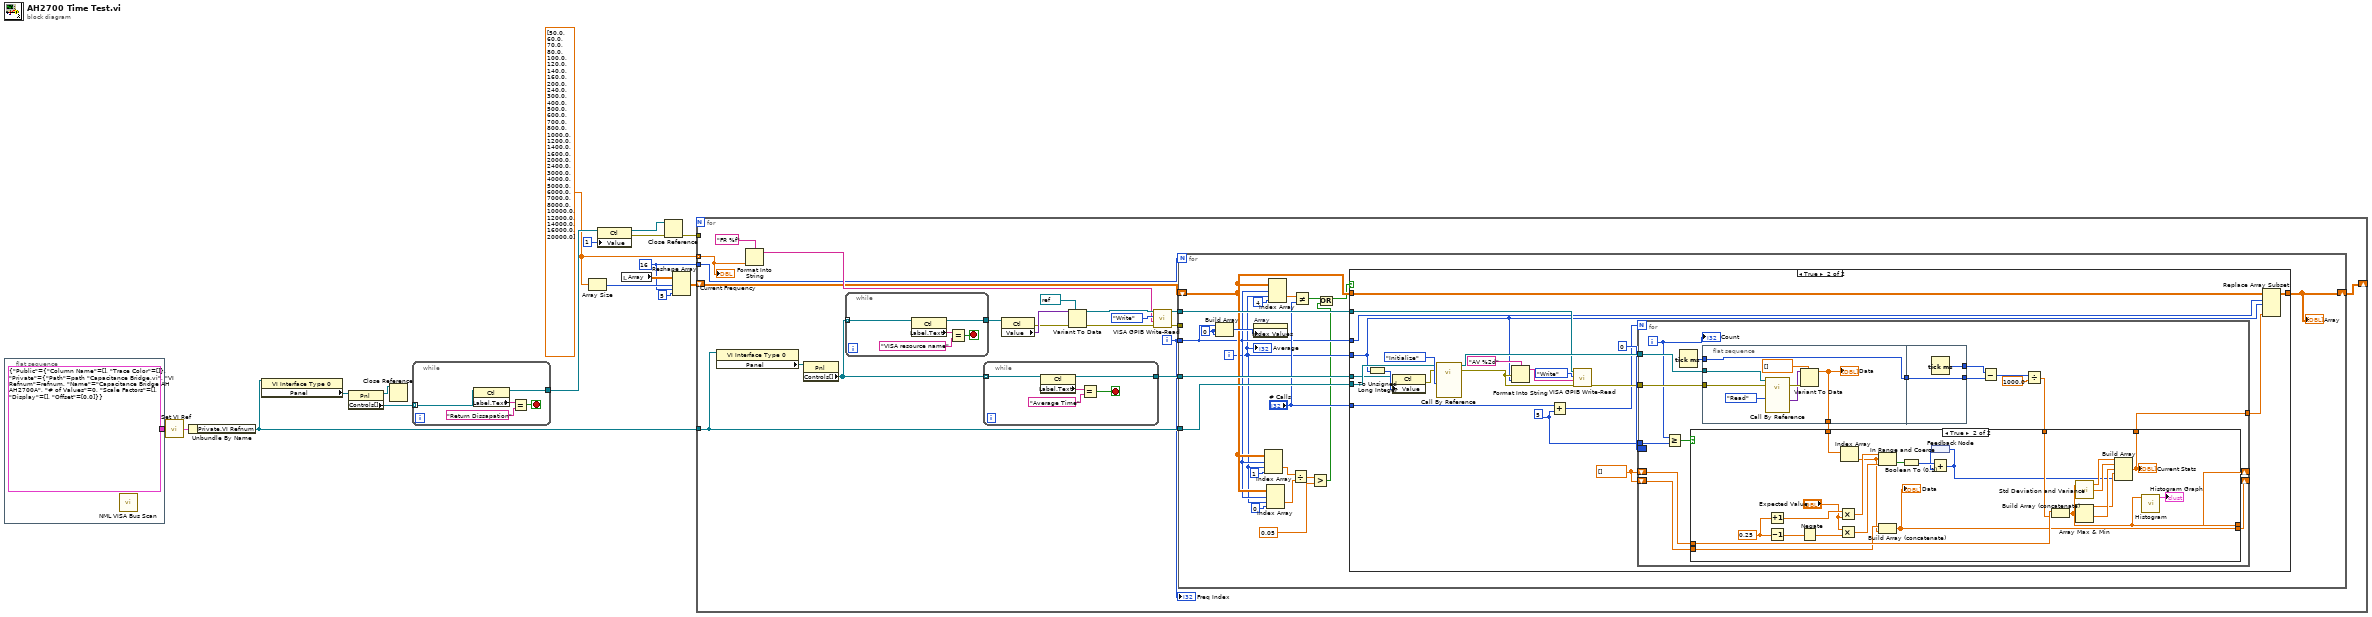
[diagram p0: block diagram]
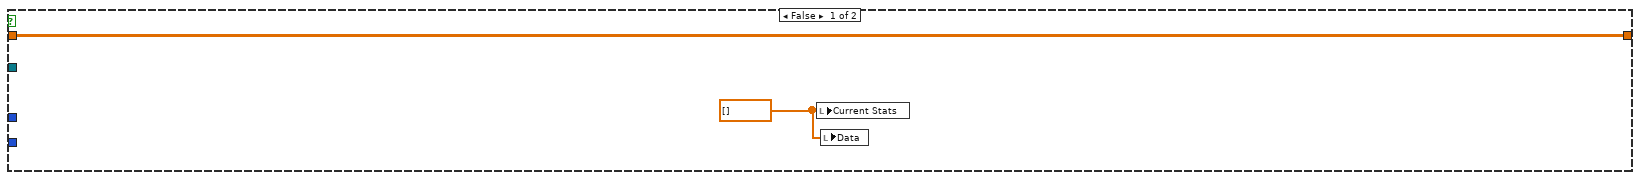
[diagram p2: hidden frame]
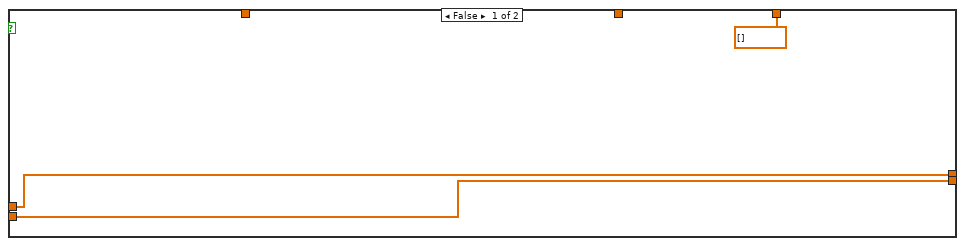
[diagram p3: hidden frame]
diagram:
  w2 = 16
  w4 = dbl[] [50.0, 60.0, 70.0, 80.0, 100.0, 120.0, 140.0, 160.0, 200.0, 240.0, 300.0, 400.0, 500.0, 600.0, 700.0, 800.0, 1000.0, 1200.0, 1400.0, 1600.0, 2000.0, 2400.0, 3000.0, 4000.0, 5000.0, 6000.0, 7000.0, 8000.0, 10000.0, 12000.0, 14000.0, 16000.0, 20000.0]
  n1 = flat-sequence {
    tunnel: [T2 {"Public"={"Column Name"=[], "Trace Color"=[]}, "Private"={"Path"=path "Capacitance Bridge.vi", "VI Refnum"=refnum, "Name"="Capacitance Bridge AH AH2700A", "# of Values"=0, "Scale Factors"=[], "Display"=[], "Offset"=[0.0]}} ("Instrument Prop In")] -> w16
    frame #0 {
      n2 = call "NML VISA Bus Scan.vi"() -> ()  [unwired: 1 in, 1 out]
    }
  }
  n3 = call "Set VI Ref.vi"("Instrument Prop In"=w16) -> ("Instrument Prop Out"=w17:T2)
  n4 = Unbundle By Name(w17) -> ("Private.VI Refnum"=w7:T5)
  n5 = property class="VI Interface Type 0"(reference=w7) -> ("Panel"=w9:refnum<vi>)  [unwired: 1 in, 2 out]
  n6 = property class="Pnl"(reference=w9) -> (reference out=w15:refnum<vi>, "Controls[]"=w10:refnum<vi>[])  [unwired: 1 in, 1 out]
  n7 = Close Reference(reference=w15) -> ()  [unwired: 1 in, 1 out]
  n8 = while {
    tunnel: w10 -> [w23] mode=indexing
    tunnel: [w19] -> w11
    stop <- w20 stop-if-true
    n9 = property class="Ctl"(reference=w23) -> (reference out=w19:refnum<vi>, "Label.Text"=w22:string)  [unwired: 1 in, 1 out]
    n10 = Equal?(x=w22, y="Return Dissapation") -> (x = y?=w20:bool)
  }
  n11 = Array Size(array=w4) -> (size(s)=w3:i32)
  n12 = property class="Ctl"(reference=w11, "Value"=1) -> (reference out=w14:refnum<vi>, error out=w13:errorcluster)  [unwired: 1 in]
  n13 = local read "Array"() -> (w6:dbl[][][])
  n14 = Close Reference(reference=w14, error in (no error)=w13) -> (error out=w8:errorcluster)
  n15 = Reshape Array(w6, w3, w2, 5 ("dimension size")) -> (w5:dbl[][][])
  n16 = for {
    tunnel: w7 -> [w41]
    tunnel: w4 -> [w31] mode=indexing
    shift-right: [w29] -> _
    shift-left: w5 -> [w25]
    tunnel: w8 -> [_]
    tunnel: w2 -> [w26]
    i -> [w24]
    n17 = property class="VI Interface Type 0"(reference=w41) -> ("Panel"=w43:refnum<vi>)  [unwired: 1 in, 2 out]
    n18 = Format Into String(format string="FR %f", w31) -> (resulting string=w30:string)  [unwired: 2 in, 1 out]
    n19 = property class="Pnl"(reference=w43) -> ("Controls[]"=w40:refnum<vi>[])  [unwired: 1 in, 2 out]
    n20 = while {
      tunnel: w40 -> [w48] mode=indexing
      tunnel: [w44] -> w39
      stop <- w45 stop-if-true
      n21 = property class="Ctl"(reference=w48) -> (reference out=w44:refnum<vi>, "Label.Text"=w47:string)  [unwired: 1 in, 1 out]
      n22 = Equal?(x=w47, y="VISA resource name") -> (x = y?=w45:bool)
    }
    n23 = while {
      tunnel: w40 -> [w53] mode=indexing
      tunnel: [w49] -> w42
      stop <- w50 stop-if-true
      n24 = property class="Ctl"(reference=w53) -> (reference out=w49:refnum<vi>, "Label.Text"=w52:string)  [unwired: 1 in, 1 out]
      n25 = Equal?(x=w52, y="Average Time") -> (x = y?=w50:bool)
    }
    n26 = property class="Ctl"(reference=w39) -> (error out=w33:errorcluster, "Value"=w38:variant)  [unwired: 1 in, 1 out]
    n27 = Variant To Data(error in=w33, type=refnum<visa-resource-name> refnum ("VISA resource name"), Variant=w38) -> (data=w36:refnum<visa-resource-name>, error out=w34:errorcluster)
    n28 = call "VISA GPIB Write-Read.vi"("error in (no error)"=w34, "Command"=w30, "Action"=enum16{"Write", "Read", "Write & Read"}."Write", "VISA resource name"=w36) -> ("error out"=w27:errorcluster, "dup VISA Session"=w28:refnum<visa-resource-name>)  [unwired: 4 in, 2 out]
    n29 = for {
      N: w26 -> [_]
      tunnel: w41 -> [w74]
      shift-right: [w65] -> w29
      shift-left: w25 -> [w62]
      tunnel: w42 -> [w73]
      tunnel: w28 -> [w72]
      tunnel: w27 -> [_]
      tunnel: w24 -> [w61]
      i -> [w60]
      w67 = 0 ("element")
      n30 = Build Array(w61, w67, w67) -> (w66:i32[])
      n31 = property on="Array" class="Arr (strict)"("Index Values"=w66) -> ()  [unwired: 2 in, 2 out]
      n32 = Index Array(array=w62, index (dim 0)=w61, index (dim 1)=w60, index (dim 2)=1 ("disabled index (col)")) -> (element=w59:dbl)
      n33 = Index Array(array=w62, index (dim 0)=w61, index (dim 1)=w60, index (dim 2)=0 ("disabled index (col)")) -> (element=w58:dbl)
      n34 = Index Array(array=w62, index (dim 0)=w61, index (dim 1)=w60, index (dim 2)=4 ("disabled index (col)")) -> (element=w70:dbl)
      n35 = Divide(x=w59, y=w58) -> (x/y=w57:dbl)
      n36 = Not Equal?(x=w70, y="# Calls") -> (x != y?=w68:bool)
      n37 = Greater?(x=w57, y=0.05) -> (0:w54:bool)
      n38 = Or(x=w68, y=w54) -> (x .or. y?=w55:bool)
      n39 = case shown="True" w55 {
        tunnel: w74 -> [_ w96]
        tunnel: "# Calls" -> [_ w93]
        tunnel: [w76 w92] -> w65
        tunnel: w62 -> [w76 w91]
        tunnel: w73 -> [_ w90]
        tunnel: w72 -> [_ w87]
        tunnel: w61 -> [_ w80]
        tunnel: w60 -> [_ w79]
        frame False {
          w75 = dbl[] [] ("Current Stats")
          n40 = local write "Current Stats"(w75) -> ()
          n41 = local write "Data"(w75) -> ()
        }
        frame True {
          w77 = 5 ("x")
          w88 = dbl[] []
          n42 = To Unsigned Long Integer(number=w79) -> (unsigned 32bit integer=w95:u32)
          n43 = property class="Ctl"(reference=w90, "Value"=w95) -> (error out=w94:errorcluster)  [unwired: 1 in, 1 out]
          n44 = call-by-ref "?"(reference=w96, error in=w94, "Action"=Instrument_Actions."Initialize") -> (reference out=w97:T5, error out=w82:errorcluster)  [unwired: 5 in, 2 out]
          n45 = Format Into String(format string="AV %2d", error in=w82, w79) -> (resulting string=w83:string)  [unwired: 1 in, 1 out]
          n46 = Add(x=w93, y=w77) -> (x+y=w78:i32)
          n47 = call "VISA GPIB Write-Read.vi"("error in (no error)"=w82, "Command"=w83, "Action"=enum16{"Write", "Read", "Write & Read"}."Write", "VISA resource name"=w87) -> ("error out"=w86:errorcluster)  [unwired: 4 in, 3 out]
          n48 = for {
            N: w78 -> [_]
            tunnel: w86 -> [w116]
            tunnel: w97 -> [w115]
            shift-right: [w111] -> _
            shift-left: w88 -> [w112]
            tunnel: [w107] -> w81
            border: i16 0 -> [_]
            shift-right: [w103] -> _
            shift-left: w88 -> [w102]
            tunnel: w77 -> [w99]
            i -> [w100]
            n49 = Greater Or Equal?(x=w100, y=w99) -> (x >= y?=w101:bool)
            n50 = Tick Count (ms)() -> (millisecond timer value=w105:u32)
            n51 = flat-sequence {
              tunnel: w116 -> [w147]
              tunnel: w115 -> [w146]
              tunnel: [w145] -> w106
              tunnel: w105 -> [w145]
              tunnel: [w144] -> w104
              tunnel: [w152] -> w113
              tunnel: [w153] -> w114
              tunnel: w106 -> [w152]
              frame #0 {
                n52 = call-by-ref "?"(reference=w146, error in=w147, "Action"=Instrument_Actions."Read") -> (error out=w151:errorcluster, "Output"=w149:variant)  [unwired: 5 in, 2 out]
                n53 = Variant To Data(error in=w151, type=dbl[] [], Variant=w149) -> (data=w144:dbl[])  [unwired: 1 out]
                "Data" <- w144
              }
              frame #1 {
                n54 = Tick Count (ms)() -> (millisecond timer value=w153:u32)
              }
            }
            n55 = Subtract(x=w114, y=w113) -> (x-y=w109:u32)
            n56 = Divide(x=w109, y=1000.0) -> (x/y=w108:dbl)
            n57 = case shown="True" w101 {
              tunnel: w112 -> [w119 w143]
              tunnel: [w119 w121] -> w111
              tunnel: w108 -> [_ w142]
              tunnel: [dbl[] [] w137] -> w107
              tunnel: w104 -> [_ w125]
              tunnel: [w118 w124] -> w103
              tunnel: w102 -> [w118 w123]
              frame False {
              }
              frame True {
                w136 = 0.25
                n58 = Increment(x=w136) -> (x+1=w133:dbl)
                n59 = Decrement(x=w136) -> (x-1=w135:dbl)
                n60 = Negate(x=w135) -> (-x=w134:dbl)
                n61 = Multiply(x=w133, y="Expected Value") -> (x*y=w132:dbl)
                n62 = Multiply(x="Expected Value", y=w134) -> (x*y=w131:dbl)
                n63 = Index Array(array=w125) -> (element=w122:dbl)  [unwired: 1 in]
                n64 = In Range and Coerce(upper limit=w132, x=w122, lower limit=w131) -> (In Range?=w129:bool)  [unwired: 1 out]
                n65 = Build Array (concatenate)(w123, w122) -> (w124:dbl[])
                "Data" <- w124
                n66 = Boolean To (0,1)(Boolean=w129) -> (0, 1=w128:i16)
                n67 = feedback #1() -> (w127:i16)
                n68 = Add(x=w128, y=w127) -> (x+y=w126:i16)
                n69 = feedback-in #1(w126) -> ()
                n70 = Build Array (concatenate)(w143, w142) -> (w121:dbl[])
                n71 = call <vilib>:"Std Deviation and Variance.vi"("X"=w121) -> ("mean"=w141:dbl, "standard deviation"=w140:dbl)  [unwired: 1 in, 1 out]
                n72 = Array Max & Min(array=w121) -> (max value=w138:dbl, min value=w139:dbl)  [unwired: 2 out]
                n73 = Build Array(w141, w140, w139, w138, w126) -> (w137:dbl[])
                "Current Stats" <- w137
                n74 = call <vilib>:"Histogram.vi"("X"=w121) -> ("Histogram Graph"=→"Histogram Graph":T1)  [unwired: 7 in, 3 out]
              }
            }
            "Count" <- w100
          }
          n75 = Replace Array Subset(array=w91, new element=w81, index (dim 0)=w80, index (dim 1)=w79) -> (w92:dbl[][][])  [unwired: 1 in]
        }
      }
      "Array" <- w65
      "Average" <- w60
    }
    "Current Frequency" <- w31
    "Freq Index" <- w24
  }
